vi "autoDrive.vi"(0 "Distance to Travel":dbl=-4.0) -> (2 "finished?":bool, 3 "left speed":dbl, 4 "right speed":dbl)   [LabVIEW 2013]
doc: "Will drive the robot at a specified speed for a specified distance. Pretty simple."
uses:
  typedefs/subStates.ctl
  typedefs/fg_typedef.ctl
  <vilib>/addons/control/pid/pid.llb/PID (DBL).vi
  <vilib>/addons/control/pid/NI_PID_pid.lvlib
panel:
  out "leftRate":dbl
  out "rightRate":dbl
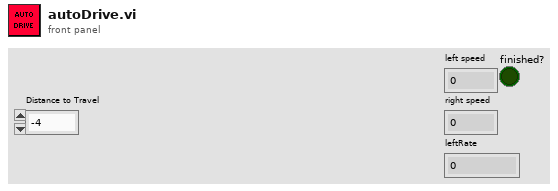
[diagram p1: front panel]
types:
  T1 = cluster{"proportional gain (Kc)":dbl, "integral time (Ti, min)":dbl, "derivative time (Td, min)":dbl}
  T2 = typedef "fg_typedef.ctl" = enum16{"Get", "Set"}
  T3 = typedef "subStates.ctl" = enum16{"null", "wait", "driver control", "auto", "manual override", "hold position", "rotate", "pickup", "pass", "load", "goto shoot", "shoot high goal", "shoot low goal", "cancel arm", "cancel shooter", "end", "test"}
  T4 = typedef "WPI_EncoderDevRef.ctl" = cluster{"DevStatus":errorcluster, "EncoderIndex":T5, "CounterIndex":T6, "DistancePerCount":dbl, "Decoding Type":T7}
  T5 = typedef "FPGA_EncoderIdx.ctl" = enum8{"Enc 0", "Enc 1", "Enc 2", "Enc 3", "Invalid"}
  T6 = typedef "FPGA_CounterCtrSystemIndex.ctl" = enum8{"Ctr 0", "Ctr 1", "Ctr 2", "Ctr 3", "Ctr 4", "Ctr 5", "Ctr 6", "Ctr 7", "Invalid"}
  T7 = typedef "WPI_EncoderType.ctl" = enum16{"1x", "2x", "4x"}
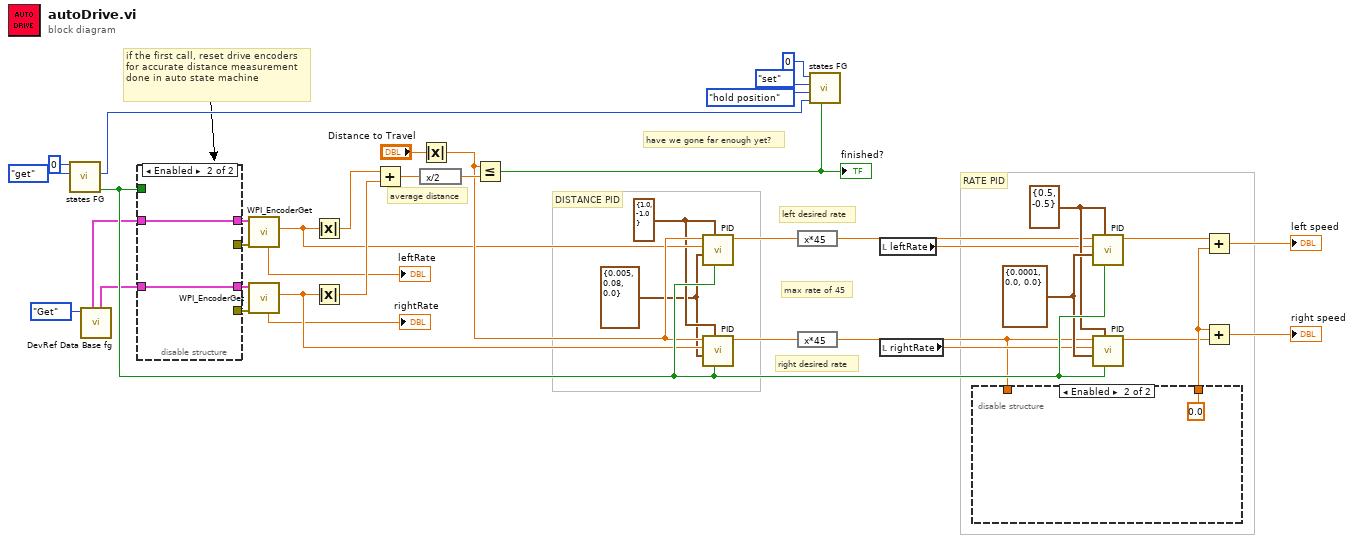
[diagram p0: block diagram]
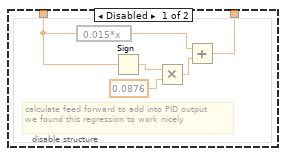
[diagram p2: hidden frame]
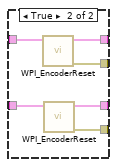
[diagram p4: hidden frame]
diagram:
  w11 = cluster{"output high":dbl, "output low":dbl} {"output high"=1.0, "output low"=-1.0} ("output range")
  w10 = T1 {"proportional gain (Kc)"=0.005, "integral time (Ti, min)"=0.08, "derivative time (Td, min)"=0.0} ("PID gains")
  w16 = T1 {"proportional gain (Kc)"=0.0001, "integral time (Ti, min)"=0.0, "derivative time (Td, min)"=0.0} ("PID gains")
  w5 = cluster{"output high":dbl, "output low":dbl} {"output high"=0.5, "output low"=-0.5} ("output range")
  # "RATE PID"
  # "DISTANCE PID"
  # "max rate of 45"
  # "left desired rate"
  # "right desired rate"
  # "if the first call, reset drive encoders for accurate distance measurement\ndone in auto state machine"
  # "have we gone far enough yet?"
  # "average distance"
  n1 = call "states FG.vi"("menu (get)"=enum16{"set", "get"}."get", "Loop ID"=0) -> ("first call?"=w40:bool, "state # out"=w24:i32)  [unwired: 6 in, 2 out]
  n2 = call "DevRef Data Base fg.vi"("Menu"=fg_typedef."Get") -> ("right drive encoder"=w18:T4, "left drive encoder"=w19:T4)  [unwired: 3 in, 4 out]
  n3 = disable-structure shown="Enabled" {
    disable-tunnel: w19 -> [w47 w57]
    disable-tunnel: w18 -> [w46 w56]
    disable-tunnel: [w45 _] -> w32
    disable-tunnel: [w44 w57] -> w31
    disable-tunnel: [w43 w56] -> w30
    disable-tunnel: [w42 _] -> w29
    disable-tunnel: w40 -> [w41 _]
    frame Disabled {
      n4 = case shown="False" w41 {
        tunnel: w47 -> [w49 w54]
        tunnel: w46 -> [w48 w52]
        tunnel: [_ w55] -> w45
        tunnel: [w49 w53] -> w44
        tunnel: [w48 w51] -> w43
        tunnel: [_ w50] -> w42
        frame False {
        }
        frame True {
          n5 = call <vilib>:"WPI_EncoderReset.vi"("EncoderDevRef"=w54) -> ("error out"=w55:errorcluster, "EncoderDevRef"=w53:T4)  [unwired: 9 in]
          n6 = call <vilib>:"WPI_EncoderReset.vi"("EncoderDevRef"=w52) -> ("error out"=w50:errorcluster, "EncoderDevRef"=w51:T4)  [unwired: 9 in]
        }
      }
    }
    frame Enabled {
    }
  }
  n7 = call <vilib>:"WPI_EncoderGet.vi"("error in (no error)"=w32, "EncoderDevRef"=w31) -> ("Distance"=w22:dbl, "Rate"=→"leftRate":dbl)  [unwired: 4 in, 4 out]
  n8 = call <vilib>:"WPI_EncoderGet.vi"("error in (no error)"=w29, "EncoderDevRef"=w30) -> ("Distance"=w21:dbl, "Rate"=→"rightRate":dbl)  [unwired: 4 in, 4 out]
  n9 = Absolute Value(x=w22) -> (abs(x)=w26:dbl)
  n10 = Absolute Value(x=w21) -> (abs(x)=w25:dbl)
  n11 = Add(x=w26, y=w25) -> (x+y=w38:dbl)
  n12 = expression code="x/2"(w38) -> (w37:dbl)
  n13 = Absolute Value(x="Distance to Travel") -> (abs(x)=w23:dbl)
  n14 = Less Or Equal?(x=w23, y=w37) -> (x <= y?=w35:bool)
  "finished?" <- w35
  n15 = call-poly <vilib>:"PID.vi"("reinitialize? (F)"=w40, "output range"=w11, "PID gains"=w10, "process variable"=w22, "setpoint"=w23) -> ("output"=w13:dbl)  [unwired: 5 in, 1 out]
  n16 = call-poly <vilib>:"PID.vi"("reinitialize? (F)"=w40, "output range"=w11, "PID gains"=w10, "process variable"=w21, "setpoint"=w23) -> ("output"=w12:dbl)  [unwired: 5 in, 1 out]
  n17 = expression code="x*45"(w13) -> (w2:dbl)
  n18 = expression code="x*45"(w12) -> (w1:dbl)
  n19 = call "states FG.vi"("exit in"=w35, "state # in"=w24, "subState in"=subStates."hold position", "menu (get)"=enum16{"set", "get"}."set", "Loop ID"=0) -> ()  [unwired: 3 in, 4 out]
  n20 = local read "leftRate"() -> (w4:dbl)
  n21 = local read "rightRate"() -> (w3:dbl)
  n22 = disable-structure shown="Enabled" {
    disable-tunnel: [w63 0.0] -> w17
    disable-tunnel: w1 -> [w58 _]
    frame Disabled {
      # "calculate feed forward to add into PID output\nwe found this regression to work nicely"
      n23 = expression code="0.015*x"(w58) -> (w62:dbl)
      n24 = Sign(1:w58) -> (0:w59:dbl)
      n25 = Multiply(x=w59, y=0.0876) -> (x*y=w61:dbl)
      n26 = Add(x=w62, y=w61) -> (x+y=w63:dbl)
    }
    frame Enabled {
    }
  }
  n27 = call-poly <vilib>:"PID.vi"("reinitialize? (F)"=w40, "output range"=w5, "PID gains"=w16, "process variable"=w4, "setpoint"=w2) -> ("output"=w15:dbl)  [unwired: 5 in, 1 out]
  n28 = call-poly <vilib>:"PID.vi"("reinitialize? (F)"=w40, "output range"=w5, "PID gains"=w16, "process variable"=w3, "setpoint"=w1) -> ("output"=w14:dbl)  [unwired: 5 in, 1 out]
  n29 = Add(x=w15, y=w17) -> (x+y=→"left speed":dbl)
  n30 = Add(x=w17, y=w14) -> (x+y=→"right speed":dbl)
